vi "REFS.vi"() -> ()   [LabVIEW 2019]
panel:
  in  "Progress":refnum<vi>
  in  "XYGraph":refnum<vi>
  in  "scrollbar":refnum<vi>
  in  "Pixel":refnum<vi>
  in  "Wavelength":refnum<vi>
  in  "offset":refnum<vi>
  in  "amplitude":refnum<vi>
  in  "raw phase":refnum<vi>
  in  "output phase":refnum<vi>
  in  "transmission":refnum<vi>
  in  "IntGraph":refnum<vi>
  in  "Task":refnum<vi>
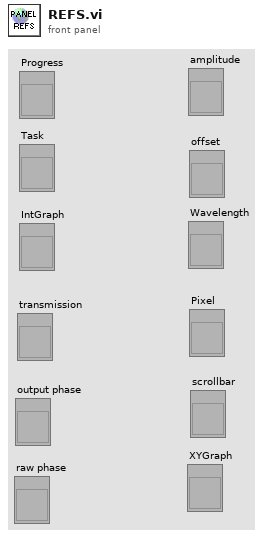
[diagram p1: front panel]
diagram:
